vi "Conection Hardware.vi"(8 "error in (no error)":errorcluster, 10 "Caracter Servicio":string="b", 11 "Hardware in":refnum<class "Hardware.lvclass">) -> (0 "error out":errorcluster, 3 "Hardware out":refnum<class "Hardware.lvclass">)   [LabVIEW 2020, in "Hardware.lvlib" / "Hardware.lvclass"]
uses:
  Hardware.lvclass
  <vilib>/Instr/_visa.llb/VISA Configure Serial Port (Instr).vi
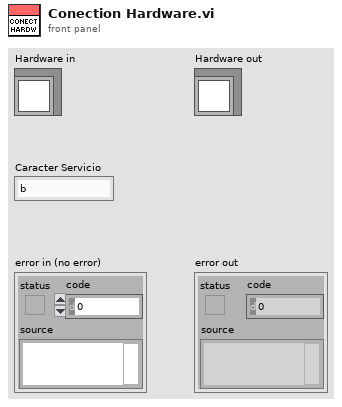
[diagram p1: front panel]
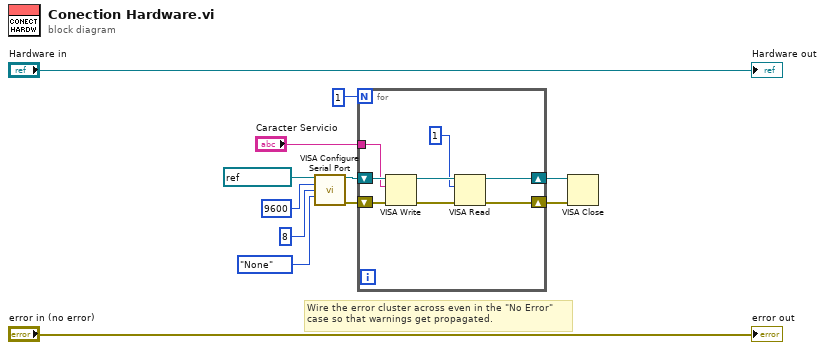
[diagram p0: block diagram]
diagram:
  # "Wire the error cluster across even in the \"No Error\"\ncase so that warnings get propagated."
  n1 = call-poly "VISA Configure Serial Port"("VISA resource name"=refnum<visa-resource-name> "COM10" ("Serial"), "baud rate (9600)"=u32 9600, "data bits (8)"=u16 8, "parity (0:none)"=enum16{"None", "Odd", "Even", "Mark", "Space"}."None") -> ("VISA resource name out"=w4:refnum<visa-resource-name>, "error out"=w3:errorcluster)  [unwired: 10 in]
  n2 = for {
    N: 1 -> [_]
    shift-right: [w20] -> w10
    shift-left: w4 -> [w18]
    shift-right: [w19] -> w9
    shift-left: w3 -> [w17]
    tunnel: "Caracter Servicio" -> [w13]
    n3 = VISA Write(VISA resource name=w18, write buffer=w13, error in (no error)=w17) -> (VISA resource name out=w16:refnum<visa-resource-name>, error out=w15:errorcluster)  [unwired: 1 out]
    n4 = VISA Read(VISA resource name=w16, byte count=u32 1, error in (no error)=w15) -> (VISA resource name out=w20:refnum<visa-resource-name>, error out=w19:errorcluster)  [unwired: 2 out]
  }
  n5 = VISA Close(VISA resource name=w10, error in (no error)=w9) -> ()  [unwired: 1 out]
  "error out" <- "error in (no error)"
  "Hardware out" <- "Hardware in"
